vi "Begin routeguide_RouteGuide_RecordRoute.vi"(8 "error in":errorcluster, 11 "gRPC ID":T1) -> (0 "error out":errorcluster, 2 "Call Id Out":T1, 3 "gRPC ID out":T1)   [LabVIEW 2019, in "route_guide_client.lvlib"]
uses:
  route_guide_client.lvlib
  <vilib>/gRPC/LabVIEW gRPC Library/Server API/typeDefs/grpcId.ctl
  <vilib>/gRPC/LabVIEW gRPC Library/gprc-lvsupport-release.lvlib
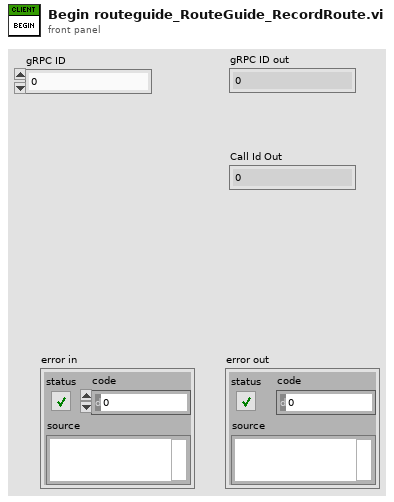
[diagram p1: front panel]
types:
  T1 = typedef "gprc-lvsupport-release.lvlib/grpcId.ctl" = u64
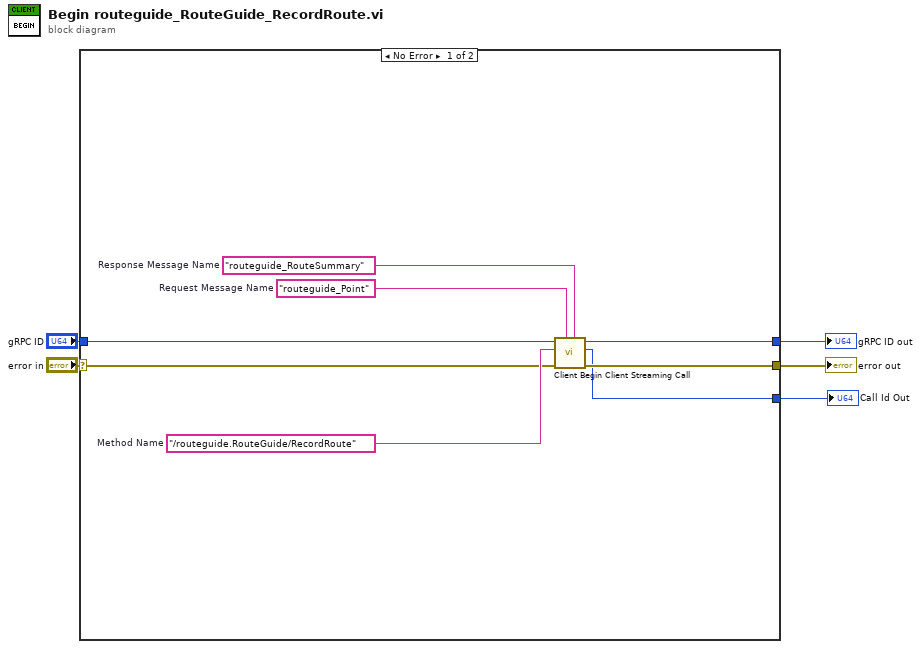
[diagram p0: block diagram]
diagram:
  n1 = case shown="No Error" "error in" {
    selector: "error in" -> [w10 w14]
    tunnel: [w9 w14] -> w4
    tunnel: "gRPC ID" -> [w8 w15]
    tunnel: [w7 w15] -> w2
    tunnel: [w6 _] -> w1
    frame No Error {
      w11 = "routeguide_RouteSummary"  # Response Message Name
      w12 = "routeguide_Point"  # Request Message Name
      w13 = "/routeguide.RouteGuide/RecordRoute"  # Method Name
      n2 = call <vilib>:"Client Begin Client Streaming Call.vi"("Response Message Name"=w11, "Request Message Name"=w12, "error in (no error)"=w10, "Method Name"=w13, "Client Ref"=w8) -> ("error out"=w9:errorcluster, "Call Id Out"=w6:T1, "Client Ref Out"=w7:T1)  [unwired: 4 in]
    }
    frame Error {
    }
  }
  "error out" <- w4
  "gRPC ID out" <- w2
  "Call Id Out" <- w1
